vi "ReadDAC_1212(Host).vi"(3 "error in (no error)":errorcluster, 4 "Address":u8 max=31 format="%.0x", 5 "Selected DAC":u8(ring)=22 items=["DAC0 (A)", "DAC1 (B)"], 6 "FPGA Interface In":refnum<k20>) -> (0 "error out":errorcluster, 1 "ReadDataI2c":fxp<+,8,8>, 2 "FPGA Interface Out":refnum<k20>)   [LabVIEW 2018]
uses:
  <vilib>/Utility/error.llb/Error Cluster From Error Code.vi
  <vilib>/rvi/errors/niLvFpgaAdjustHostInterfaceError.vi
  <vilib>/rvi/interface/nirviReadWriteControl/nirviReadWriteControl.xnode
  NiFpgaLv.dll
  <vilib>/rvi/interface/Simulation/niFpgaSimulationCallBeginRW.vi
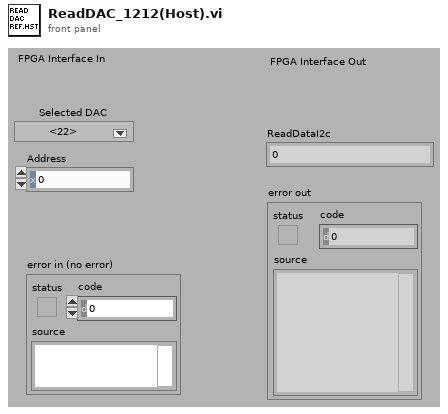
[diagram p1: front panel]
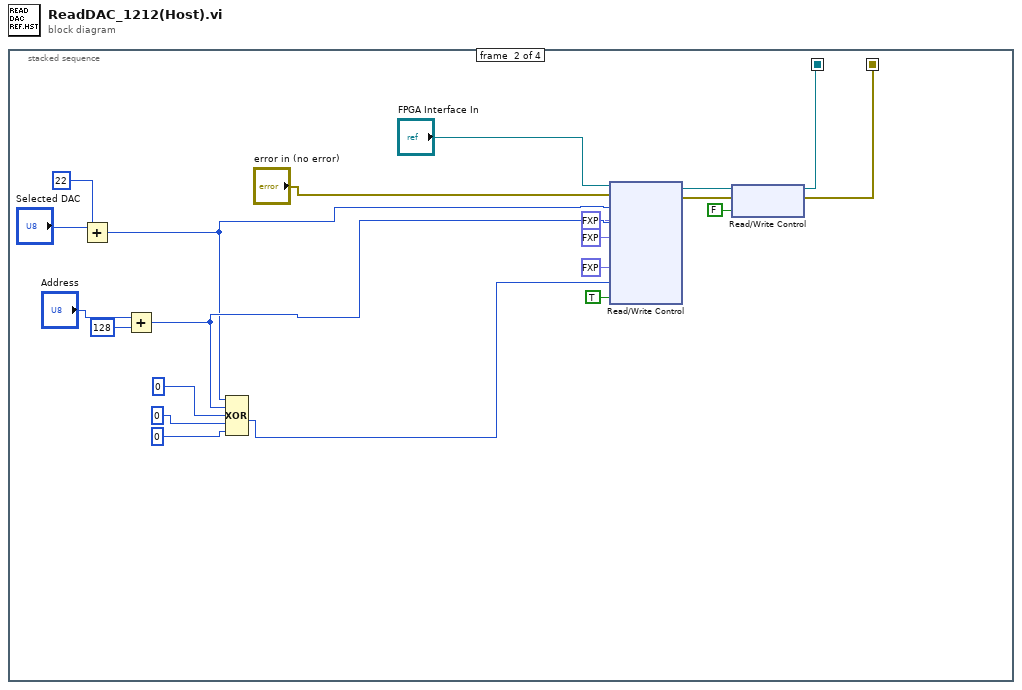
[diagram p0: block diagram]
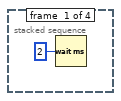
[diagram p2: hidden frame]
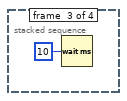
[diagram p3: hidden frame]
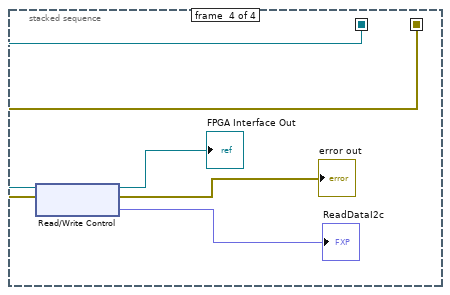
[diagram p4: hidden frame]
diagram:
  n1 = stacked-sequence {
    seq-local: [_ w6 _ _] -> [_ _ _ w28]
    seq-local: [_ w5 _ _] -> [_ _ _ w27]
    frame #0 {
      n2 = Wait (ms)(milliseconds to wait=u32 2) -> ()  [unwired: 1 out]
    }
    frame #1 {
      n3 = Add(x="Selected DAC", y=u8 22) -> (x+y=w4:u8)
      n4 = Add(x="Address", y=u8 128) -> (x+y=w14:u8)
      n5 = Compound Arithmetic op=XOR(w4, w14, u8 0 ("value"), u8 0, u8 0) -> (w10:u8)
      n6 = xnode "Read/Write Control"("FPGA VI Reference In"="FPGA Interface In", "error in"="error in (no error)", "DataI2c0"=w4, "DataI2c1"=w14, "DataI2c2"=fxp<+,8,8> 0.0, "DataI2c3"=fxp<+,8,8> 0.0, "DataI2c4"=fxp<+,8,8> 0.0, "DataI2c5"=w10, "StartRDI2c"=TRUE) -> ("FPGA VI Reference Out"=w8:refnum<k20>, "error out"=w7:errorcluster)
      n7 = xnode "Read/Write Control"("FPGA VI Reference In"=w8, "error in"=w7, "StartRDI2c"=FALSE) -> ("FPGA VI Reference Out"=w6:refnum<k20>, "error out"=w5:errorcluster)
    }
    frame #2 {
      n8 = Wait (ms)(milliseconds to wait=u32 10) -> ()  [unwired: 1 out]
    }
    frame #3 {
      n9 = xnode "Read/Write Control"("FPGA VI Reference In"=w28, "error in"=w27) -> ("FPGA VI Reference Out"=→"FPGA Interface Out":refnum<k20>, "error out"=→"error out":errorcluster, "ReadDataI2c"=→"ReadDataI2c":fxp<+,8,8>)
    }
  }
